vi "conditionally open vi ref.vi"(6 "call chain index (1)":i32=1, 8 "error in (no error)":errorcluster, 11 "vi ref in":refnum<vi>) -> (0 "error out":errorcluster, 3 "vi ref out":refnum<vi>, 5 "new ref?":bool)   [LabVIEW 2024, in "controls manager.lvlib"]
uses:
  controls manager.lvlib
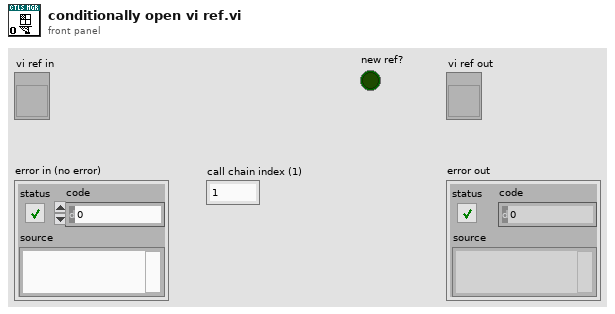
[diagram p1: front panel]
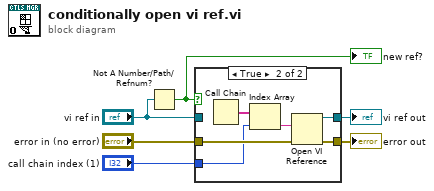
[diagram p0: block diagram]
diagram:
  n1 = Not A Number/Path/Refnum?(number/path/refnum="vi ref in") -> (NaN/Path/Refnum?=w3:bool)
  "new ref?" <- w3
  n2 = case shown="True" w3 {
    tunnel: [w8 w13] -> w4
    tunnel: "vi ref in" -> [w8 _]
    tunnel: [w7 w12] -> w2
    tunnel: "error in (no error)" -> [w7 w11]
    tunnel: "call chain index (1)" -> [_ w10]
    frame False {
    }
    frame True {
      n3 = Call Chain() -> (call chain=w14:string[])
      n4 = Index Array(array=w14, index=w10) -> (element=w9:string)
      n5 = Open VI Reference(vi path=w9, error in (no error)=w11) -> (vi reference=w13:refnum<vi>, error out=w12:errorcluster)  [unwired: 4 in]
    }
  }
  "vi ref out" <- w4
  "error out" <- w2
